vi "DAQ 1SDI v06.vi"() -> ()   [LabVIEW 2013]
uses:
  <instrlib>/niScope/Controls/niScope vertical coupling.ctl
  Strict Type Defs/type_meas_enum.ctl
panel:
  out "Waveform Graph":waveform(dbl)[](graph)
  in  "minSamples":i32=1000000 caption="numSamples"
  in  "number of files":i32=5
  in  "maxSamples":i32=1000000 caption="numSamples"
  in  "Run":string="1"
  in  "Name root":string="test"
  in  "Type of\nmeasurement":T1=enum."x"
  in  "File location":path=path "C:/ni-rt/LabVIEW Data/testing"
  in  "channel parms":T3={"input impedance"=2, "maximum input frequency"=7000000.0, "vertical coupling"=1, "probe attenuation"=1.0, "vertical range"=0.5, "vertical offset"=0.0, "channel enabled"=TRUE} {"input impedance" items=["1 mega ohm"=0, "50 ohms"=2]; "vertical coupling" items=["AC", "DC", "Ground"]}
  in  "Take Data":bool
  in  "stop":bool
  out "error out":errorcluster
  in  "reference position":dbl=50.0
  in  "error in":errorcluster
  in  "resource names":T4={"resource 1"="Dev2", "resource 2"="Dev3"}
  in  "min sample rate":dbl=100000000.0
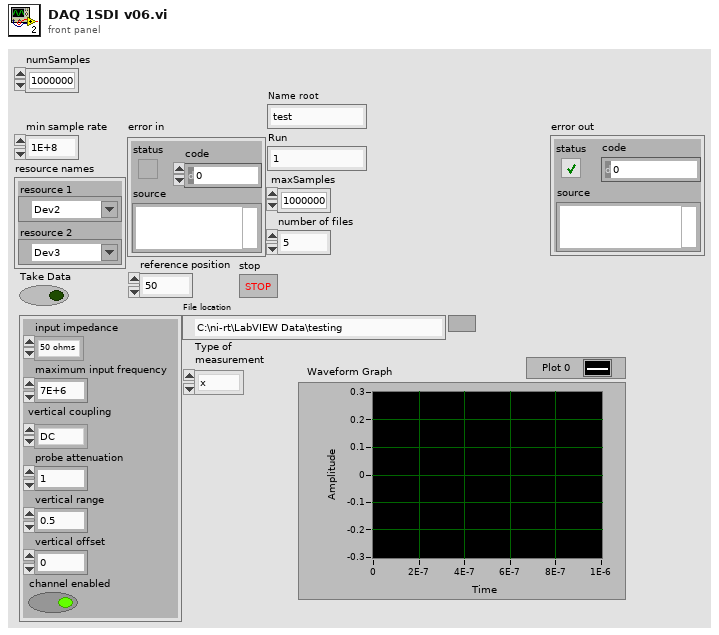
[diagram p1: front panel]
types:
  T1 = typedef "type_meas_enum.ctl" = enum16{"shot", "x", "p", "electronic"}
  T2 = typedef "niScope vertical coupling.ctl" = i32
  T3 = cluster{"input impedance":u32, "maximum input frequency":dbl, "vertical coupling":T2, "probe attenuation":dbl, "vertical range":dbl, "vertical offset":dbl, "channel enabled":bool}
  T4 = cluster{"resource 1":refnum<k15>, "resource 2":refnum<k15>}
  T5 = cluster{"instrument handle out 0":refnum<k15>, "instrument handle out 1":refnum<k15>}
  T6 = cluster{"instrument handle out":refnum<k15>, "instrument handle out":refnum<k15>}
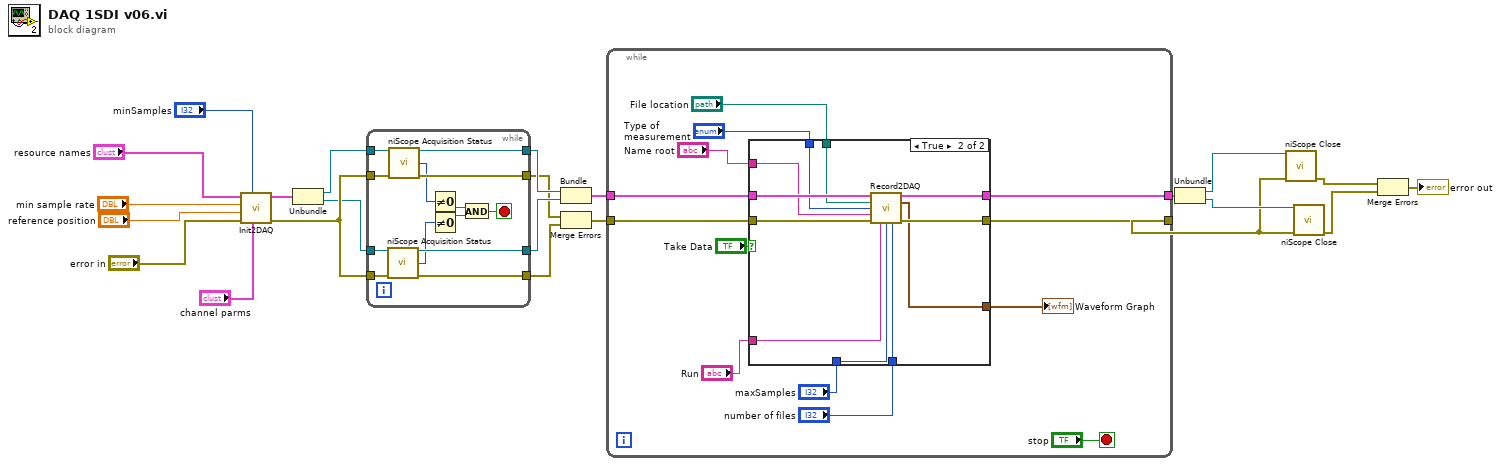
[diagram p0: block diagram]
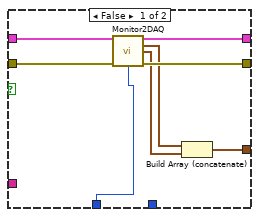
[diagram p2: hidden frame]
diagram:
  n1 = call "Init2DAQ.vi"("channel parms"="channel parms", "min record length"="minSamples", "error in"="error in", "reference position"="reference position", "min sample rate"="min sample rate", "resource names"="resource names") -> ("error out"=w11:errorcluster, "instrument out"=w10:T5)  [unwired: 4 in]
  n2 = Unbundle(w10) -> ("instrument handle out 0"=w9:refnum<k15>, "instrument handle out 1"=w8:refnum<k15>)
  n3 = while {
    tunnel: w9 -> [w35]
    tunnel: w11 -> [w34]
    tunnel: w8 -> [w32]
    tunnel: w11 -> [w29]
    tunnel: [w36] -> w6
    tunnel: [w33] -> w3
    tunnel: [w31] -> w5
    tunnel: [w30] -> w2
    stop <- w24 stop-if-true
    n4 = call <instrlib>:"niScope Acquisition Status.vi"("instrument handle"=w32, "error in"=w29) -> ("instrument handle out"=w31:refnum<k15>, "acquisition status"=w28:i32, "error out"=w30:errorcluster)  [unwired: 11 in]
    n5 = call <instrlib>:"niScope Acquisition Status.vi"("instrument handle"=w35, "error in"=w34) -> ("instrument handle out"=w36:refnum<k15>, "acquisition status"=w27:i32, "error out"=w33:errorcluster)  [unwired: 11 in]
    n6 = Not Equal To 0?(x=w27) -> (x != 0?=w26:bool)
    n7 = Not Equal To 0?(x=w28) -> (x != 0?=w25:bool)
    n8 = And(x=w26, y=w25) -> (x .and. y?=w24:bool)
  }
  n9 = Bundle("instrument handle out"=w6, "instrument handle out"=w5) -> (w7:T6)  [unwired: 1 in]
  n10 = Merge Errors(w3, w2) -> (w4:errorcluster)
  n11 = while {
    tunnel: w7 -> [w48]
    tunnel: w4 -> [w47]
    tunnel: [w44] -> w19
    tunnel: [w45] -> w16
    stop <- "stop" stop-if-true
    n12 = case shown="True" "Take Data" {
      tunnel: w48 -> [w57 w68]
      tunnel: w47 -> [w56 w67]
      tunnel: [w54 w65] -> w44
      tunnel: [w55 w66] -> w45
      tunnel: "number of files" -> [_ w64]
      tunnel: "maxSamples" -> [w53 w63]
      tunnel: "Run" -> [_ w62]
      tunnel: "Name root" -> [_ w61]
      tunnel: "Type of\nmeasurement" -> [_ w60]
      tunnel: "File location" -> [_ w59]
      tunnel: [w52 w58] -> w37
      frame False {
        n13 = call "Monitor2DAQ.vi"("instrument in"=w57, "error in"=w56, "numSamples"=w53) -> ("instrument out"=w54:T5, "wfm 1"=w51:waveform(dbl)[], "wfm 2"=w50:waveform(dbl)[], "error out"=w55:errorcluster)  [unwired: 9 in]
        n14 = Build Array (concatenate)(w51, w50) -> (w52:waveform(dbl)[])
      }
      frame True {
        n15 = call "Record2DAQ.vi"("instrument in"=w68, "File location"=w59, "Type of\nmeasurement"=w60, "Name root"=w61, "error in"=w67, "Run"=w62, "numSamples"=w63, "number of files"=w64) -> ("instrument out"=w65:T5, "waveform"=w58:waveform(dbl)[], "error out"=w66:errorcluster)  [unwired: 3 in, 2 out]
      }
    }
    "Waveform Graph" <- w37
  }
  n16 = Unbundle(w19) -> ("instrument handle out 0"=w18:refnum<k15>, "instrument handle out 1"=w17:refnum<k15>)
  n17 = call <instrlib>:"niScope Close.vi"("instrument handle"=w18, "error in"=w16) -> ("error out"=w15:errorcluster)  [unwired: 13 in]
  n18 = call <instrlib>:"niScope Close.vi"("instrument handle"=w17, "error in"=w16) -> ("error out"=w14:errorcluster)  [unwired: 13 in]
  n19 = Merge Errors(w15, w14) -> (→"error out":errorcluster)
